vi "Teleop - Pincher Control.vi"(10 "Joystick 1 Buttons":bool[](array[boolean]), 11 "Joystick 0 Buttons":bool[](array[boolean])) -> ()   [LabVIEW 2017]
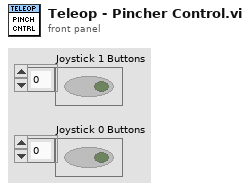
[diagram p1: front panel]
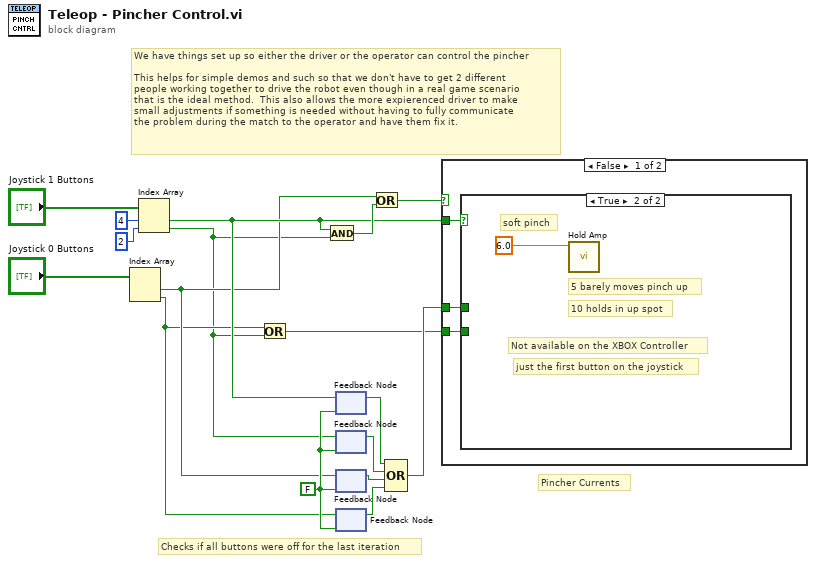
[diagram p0: block diagram]
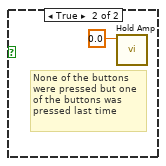
[diagram p3: hidden frame]
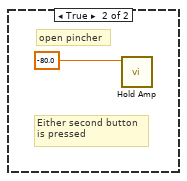
[diagram p4: hidden frame]
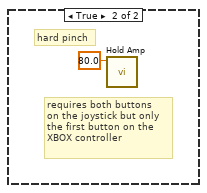
[diagram p5: hidden frame]
diagram:
  w15 = FALSE
  # "Checks if all buttons were off for the last iteration"
  # "We have things set up so either the driver or the operator can control the pincher\n\nThis helps for simple demos and such so that we don't have to get 2 different\npeople working together to drive the robot even though in a real game scenario\nthat is the ideal method.  This also allows the more expierenced driver to make \nsmall adjustments if something is needed without having to fully communicate\nthe problem during the match to the operator and have them fix it."
  # "Pincher Currents"
  n1 = Index Array(array="Joystick 0 Buttons") -> (element #1=w4:bool, element #2=w2:bool)  [unwired: 2 in]
  n2 = Index Array(array="Joystick 1 Buttons", index #1=4 ("index"), index #2=2 ("index")) -> (element #1=w5:bool, element #2=w1:bool)
  n3 = Or(x=w2, y=w1) -> (x .or. y?=w3:bool)
  n4 = And(x=w5, y=w1) -> (x .and. y?=w13:bool)
  n5 = feedback #1(w15) -> (w7:bool)
  n6 = feedback-in #1(w5) -> ()
  n7 = feedback #2(w15) -> (w6:bool)
  n8 = feedback-in #2(w1) -> ()
  n9 = feedback #3(w15) -> (w10:bool)
  n10 = feedback-in #3(w4) -> ()
  n11 = feedback #4(w15) -> (w9:bool)
  n12 = feedback-in #4(w2) -> ()
  n13 = Or(x=w4, y=w13) -> (x .or. y?=w14:bool)
  n14 = Compound Arithmetic op=OR(w7, w6, w10, w9) -> (w8:bool)
  n15 = case shown="False" w14 {
    tunnel: w5 -> [w20 _]
    tunnel: w8 -> [w19 _]
    tunnel: w3 -> [w18 _]
    frame False {
      n16 = case shown="True" w20 {
        tunnel: w19 -> [w22 _]
        tunnel: w18 -> [w21 _]
        frame False {
          n17 = case shown="False" w21 {
            tunnel: w22 -> [w23 _]
            frame False {
              n18 = case shown="False" w23 {
                frame False {
                  # "no buttons\npressed this\ntime or\nlast time\ndo nothing"
                }
                frame True {
                  # "None of the buttons\nwere pressed but one\nof the buttons was\npressed last time"
                  n19 = call "Hold Amp.vi"("Setpoint"=0.0) -> ()  [unwired: 10 in, 1 out]
                }
              }
            }
            frame True {
              # "Either second button\nis pressed"
              # "open pincher"
              n20 = call "Hold Amp.vi"("Setpoint"=-80.0 ("5")) -> ()  [unwired: 10 in, 1 out]
            }
          }
        }
        frame True {
          # "just the first button on the joystick"
          # "Not available on the XBOX Controller"
          # "10 holds in up spot"
          # "5 barely moves pinch up"
          # "soft pinch"
          n21 = call "Hold Amp.vi"("Setpoint"=6.0 ("4")) -> ()  [unwired: 10 in, 1 out]
        }
      }
    }
    frame True {
      # "requires both buttons\non the joystick but only\nthe first button on the\nXBOX controller"
      # "hard pinch"
      n22 = call "Hold Amp.vi"("Setpoint"=80.0 ("Both")) -> ()  [unwired: 10 in, 1 out]
    }
  }
